vi "IterativeMove.vi"(0 "Handle":i32, 1 "IterativeMoves":i32, 3 "Axis":u32, 4 "Velocity":dbl, 5 "Threshold (mm)":dbl, 8 "Goal":dbl) -> ()   [LabVIEW 2012]
uses:
  MicroDrive.dll
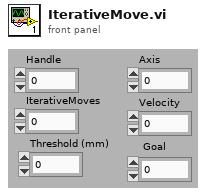
[diagram p1: front panel]
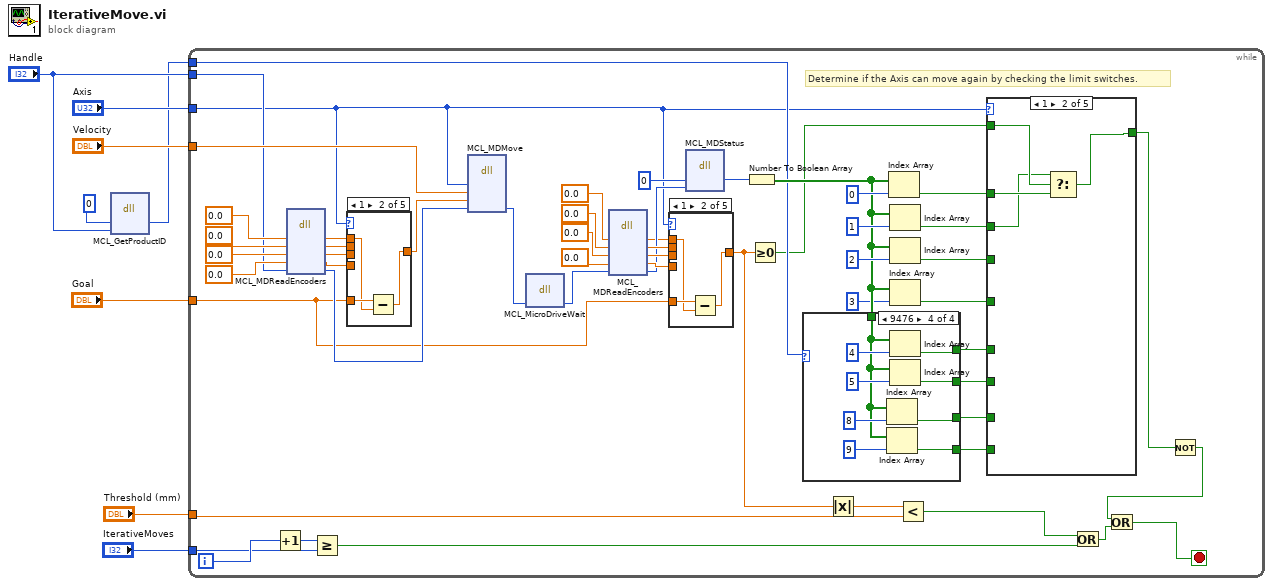
[diagram p0: block diagram]
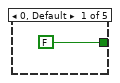
[diagram p2: hidden frame]
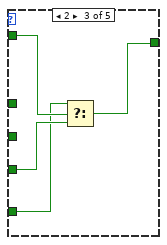
[diagram p3: hidden frame]
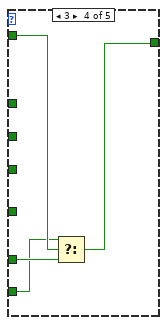
[diagram p4: hidden frame]
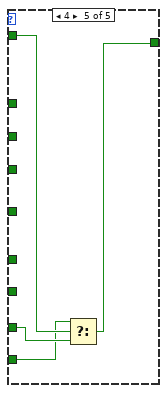
[diagram p5: hidden frame]
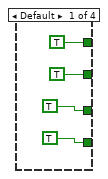
[diagram p6: hidden frame]
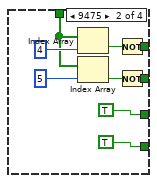
[diagram p7: hidden frame]
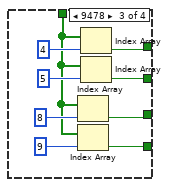
[diagram p8: hidden frame]
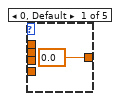
[diagram p9: hidden frame]
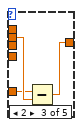
[diagram p10: hidden frame]
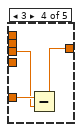
[diagram p11: hidden frame]
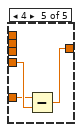
[diagram p12: hidden frame]
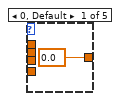
[diagram p13: hidden frame]
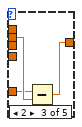
[diagram p14: hidden frame]
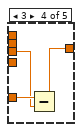
[diagram p15: hidden frame]
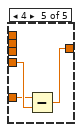
[diagram p16: hidden frame]
diagram:
  n1 = dll-call lib="C:/Users/Labview/Desktop/SRR/MicroDrive_x64/MicroDrive.dll" fn="MCL_GetProductID"("PID"=u16 0, "handle"="Handle") -> ("PID"=w3:u16)  [unwired: 4 in, 3 out]
  n2 = while {
    tunnel: "Handle" -> [w54]
    tunnel: "Axis" -> [w35]
    tunnel: "Velocity" -> [w62]
    tunnel: "Goal" -> [w45]
    tunnel: w3 -> [w36]
    tunnel: "Threshold (mm)" -> [w23]
    tunnel: "IterativeMoves" -> [w19]
    i -> [w21]
    stop <- w14 stop-if-true
    # "Determine if the Axis can move again by checking the limit switches."
    n3 = Increment(x=w21) -> (x+1=w20:i32)
    n4 = dll-call lib="C:/Users/Labview/Desktop/SRR/MicroDrive_x64/MicroDrive.dll" fn="MCL_MDReadEncoders"("m1"=0.0, "m2"=0.0, "m3"=0.0, "m4"=0.0, "handle"=w54) -> ("m1"=w13:dbl, "m2"=w57:dbl, "m3"=w56:dbl, "m4"=w55:dbl, "handle"=w53:i32)  [unwired: 3 in, 3 out]
    n5 = Greater Or Equal?(x=w20, y=w19) -> (x >= y?=w18:bool)
    n6 = case shown="1" w35 {
      tunnel: w13 -> [_ w125 _ _ _]
      tunnel: w57 -> [_ _ w130 _ _]
      tunnel: w56 -> [_ _ _ w132 _]
      tunnel: w55 -> [_ _ _ _ w136]
      tunnel: [0.0 w126 w128 w131 w134] -> w12
      tunnel: w45 -> [_ w127 w129 w133 w135]
      frame 0, Default {
      }
      frame 1 {
        n7 = Subtract(x=w127, y=w125) -> (x-y=w126:dbl)
      }
      frame 2 {
        n8 = Subtract(x=w129, y=w130) -> (x-y=w128:dbl)
      }
      frame 3 {
        n9 = Subtract(x=w133, y=w132) -> (x-y=w131:dbl)
      }
      frame 4 {
        n10 = Subtract(x=w135, y=w136) -> (x-y=w134:dbl)
      }
    }
    n11 = dll-call lib="C:/Users/Labview/Desktop/SRR/MicroDrive_x64/MicroDrive.dll" fn="MCL_MDMove"("axis"=w35, "velocity"=w62, "distance"=w12, "handle"=w53) -> ("handle"=w11:i32)  [unwired: 6 in, 3 out]
    n12 = dll-call lib="C:/Users/Labview/Desktop/SRR/MicroDrive_x64/MicroDrive.dll" fn="MCL_MicroDriveWait"("handle"=w11) -> ("handle"=w10:i32)  [unwired: 3 in, 3 out]
    n13 = dll-call lib="C:/Users/Labview/Desktop/SRR/MicroDrive_x64/MicroDrive.dll" fn="MCL_MDReadEncoders"("m1"=0.0, "m2"=0.0, "m3"=0.0, "m4"=0.0, "handle"=w10) -> ("m1"=w9:dbl, "m2"=w48:dbl, "m3"=w47:dbl, "m4"=w46:dbl, "handle"=w38:i32)  [unwired: 3 in, 3 out]
    n14 = case shown="1" w35 {
      tunnel: w9 -> [_ w112 _ _ _]
      tunnel: w48 -> [_ _ w117 _ _]
      tunnel: w47 -> [_ _ _ w119 _]
      tunnel: w46 -> [_ _ _ _ w123]
      tunnel: [0.0 w113 w115 w118 w121] -> w25
      tunnel: w45 -> [_ w114 w116 w120 w122]
      frame 0, Default {
      }
      frame 1 {
        n15 = Subtract(x=w114, y=w112) -> (x-y=w113:dbl)
      }
      frame 2 {
        n16 = Subtract(x=w116, y=w117) -> (x-y=w115:dbl)
      }
      frame 3 {
        n17 = Subtract(x=w120, y=w119) -> (x-y=w118:dbl)
      }
      frame 4 {
        n18 = Subtract(x=w122, y=w123) -> (x-y=w121:dbl)
      }
    }
    n19 = dll-call lib="C:/Users/Labview/Desktop/SRR/MicroDrive_x64/MicroDrive.dll" fn="MCL_MDStatus"("status"=u16 0, "handle"=w38) -> ("status"=w37:u16)  [unwired: 4 in, 3 out]
    n20 = Number To Boolean Array(number=w37) -> (Boolean array=w41:bool[])
    n21 = Greater Or Equal To 0?(x=w25) -> (x >= 0?=w34:bool)
    n22 = case shown="9476" w36 {
      tunnel: [TRUE w91 w96 w105] -> w29
      tunnel: w41 -> [_ w89 w97 w106]
      tunnel: [TRUE w87 w95 w104] -> w28
      tunnel: [TRUE TRUE w94 w103] -> w27
      tunnel: [TRUE TRUE w93 w102] -> w26
      frame Default {
      }
      frame 9475 {
        n23 = Index Array(array=w89, index=4) -> (element=w92:bool)
        n24 = Index Array(array=w89, index=5) -> (element=w86:bool)
        n25 = Not(x=w92) -> (.not. x?=w91:bool)
        n26 = Not(x=w86) -> (.not. x?=w87:bool)
      }
      frame 9478 {
        n27 = Index Array(array=w97, index=8) -> (element=w94:bool)
        n28 = Index Array(array=w97, index=9) -> (element=w93:bool)
        n29 = Index Array(array=w97, index=4) -> (element=w96:bool)
        n30 = Index Array(array=w97, index=5) -> (element=w95:bool)
      }
      frame 9476 {
        n31 = Index Array(array=w106, index=8) -> (element=w103:bool)
        n32 = Index Array(array=w106, index=9) -> (element=w102:bool)
        n33 = Index Array(array=w106, index=4) -> (element=w105:bool)
        n34 = Index Array(array=w106, index=5) -> (element=w104:bool)
      }
    }
    n35 = Absolute Value(x=w25) -> (abs(x)=w24:dbl)
    n36 = Index Array(array=w41, index=0) -> (element=w33:bool)
    n37 = Index Array(array=w41, index=1) -> (element=w32:bool)
    n38 = Index Array(array=w41, index=2) -> (element=w31:bool)
    n39 = Index Array(array=w41, index=3) -> (element=w30:bool)
    n40 = Less?(x=w24, y=w23) -> (x < y?=w17:bool)
    n41 = case shown="1" w35 {
      tunnel: w34 -> [_ w67 w71 w75 w79]
      tunnel: [FALSE w64 w68 w72 w76] -> w22
      tunnel: w33 -> [_ w66 _ _ _]
      tunnel: w32 -> [_ w65 _ _ _]
      tunnel: w31 -> [_ _ w70 _ _]
      tunnel: w30 -> [_ _ w69 _ _]
      tunnel: w29 -> [_ _ _ w74 _]
      tunnel: w28 -> [_ _ _ w73 _]
      tunnel: w27 -> [_ _ _ _ w78]
      tunnel: w26 -> [_ _ _ _ w77]
      frame 0, Default {
      }
      frame 1 {
        n42 = Select(t=w65, s=w67, f=w66) -> (s? t:f=w64:bool)
      }
      frame 2 {
        n43 = Select(t=w69, s=w71, f=w70) -> (s? t:f=w68:bool)
      }
      frame 3 {
        n44 = Select(t=w73, s=w75, f=w74) -> (s? t:f=w72:bool)
      }
      frame 4 {
        n45 = Select(t=w77, s=w79, f=w78) -> (s? t:f=w76:bool)
      }
    }
    n46 = Or(x=w17, y=w18) -> (x .or. y?=w16:bool)
    n47 = Not(x=w22) -> (.not. x?=w15:bool)
    n48 = Or(x=w15, y=w16) -> (x .or. y?=w14:bool)
  }
